vi "아날로그 out.vi"() -> ()   [LabVIEW 2018]
uses:
  <vilib>/DAQmx/write.llb/DAQmx Write (Analog DBL 1Chan 1Samp).vi
  <vilib>/DAQmx/create/channels.llb/DAQmx Create Channel (AO-Voltage-Basic).vi
  <vilib>/DAQmx/miscellaneous.llb/DAQmx Fill In Error Info.vi
panel:
  in  "physical channels 2":tag caption="물리적 채널"
  in  "data":dbl(knob) caption="데이터" scale=0.0..10.0
  in  "minimum value":dbl=-5.0 caption="최소값" format="%0.2f"
  in  "maximum value":dbl=5.0 caption="최대값" format="%0.2f"
  in  "name to assign":string caption="할당된 이름"
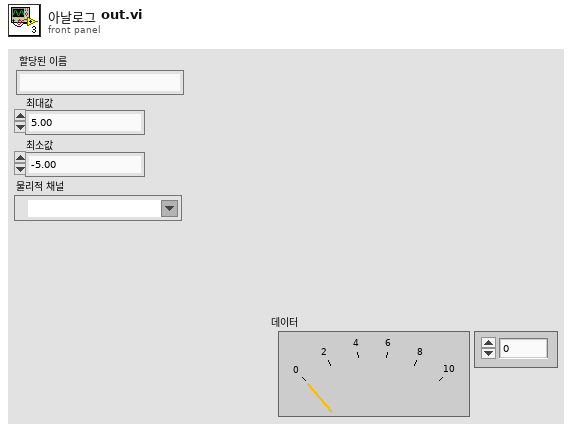
[diagram p1: front panel]
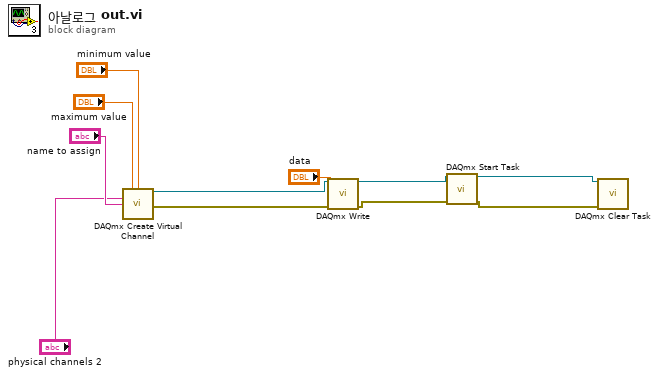
[diagram p0: block diagram]
diagram:
  n1 = call-poly <vilib>:"DAQmx Create Virtual Channel.vi"("maximum value"="maximum value", "minimum value"="minimum value", "physical channels"="physical channels 2", "name to assign"="name to assign") -> ("task out"=w8:refnum<k21>, "error out"=w7:errorcluster)  [unwired: 10 in]
  n2 = call-poly <vilib>:"DAQmx Write.vi"("task/channels in"=w8, "data"="data", "error in"=w7) -> ("task out"=w5:refnum<k21>, "error out"=w4:errorcluster)  [unwired: 10 in, 1 out]
  n3 = call <vilib>:"DAQmx Start Task.vi"("task/channels in"=w5, "error in"=w4) -> ("task out"=w3:refnum<k21>, "error out"=w2:errorcluster)  [unwired: 12 in]
  n4 = call <vilib>:"DAQmx Clear Task.vi"("task in"=w3, "error in"=w2) -> ()  [unwired: 13 in, 1 out]
